vi "Compile Routing and Faulting Config.vi"(8 "error in (no error)":errorcluster, 11 "Device Ref in":T1 format="%.0x") -> (0 "error out":errorcluster, 2 "RaF Configuration":T2, 3 "Device Ref out":T1 format="%.0x")   [LabVIEW 2017, in "Routing and Faulting System Explorer.lvlib"]
uses:
  Routing and Faulting System Explorer.lvlib
  Shared/Routing and Faulting Configuration.ctl
  Shared/Routing Channel Configuration.ctl
  Shared/Value-Connections Map.ctl
  Shared/Connection.ctl
  <vilib>/NI Veristand/Custom Device API/Custom Device Item Ref.ctl
  Shared/Constants.vi
  <vilib>/NI Veristand/Custom Device Tools/Custom Device Utility Library/NI VeriStand - Search for Item by Name.vi
  Shared/Routing and Faulting Shared.lvlib
  <vilib>/NI Veristand/Custom Device Tools/Custom Device Utility Library/Custom Device Utility Library.lvlib
  Scripting/Switch Scripting.lvlib
  <vilib>/NI VeriStand/Custom Device API/Custom Device API.lvlib
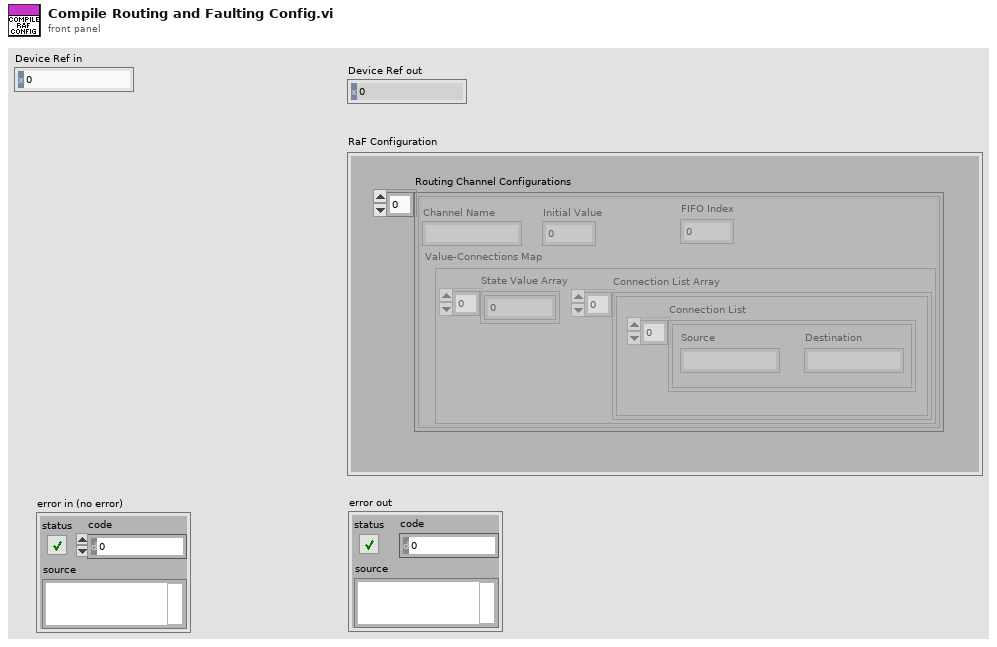
[diagram p1: front panel]
types:
  T1 = typedef "Custom Device API.lvlib/Custom Device Item Ref.ctl" = u64
  T2 = typedef "Routing and Faulting Shared.lvlib/Routing and Faulting Configuration.ctl" = cluster{"Routing Channel Configurations":T3[]}
  T3 = typedef "Routing and Faulting Shared.lvlib/Routing Channel Configuration.ctl" = cluster{"Channel Name":string, "Initial Value":dbl, "FIFO Index":i32, "Value-Connections Map":T4}
  T4 = typedef "Routing and Faulting Shared.lvlib/Value-Connections Map.ctl" = cluster{"State Value Array":i32[], "Connection List Array":cluster{"Connection List":T5[]}[]}
  T5 = typedef "Routing and Faulting Shared.lvlib/Connection.ctl" = cluster{"Source":string, "Destination":string}
  T6 = typedef "Routing and Faulting Shared.lvlib/Channel States.ctl" = T7[]
  T7 = typedef "Routing and Faulting Shared.lvlib/Routing State.ctl" = cluster{"Name":string, "Description":string, "Value":i32, "Connection List":T5[]}
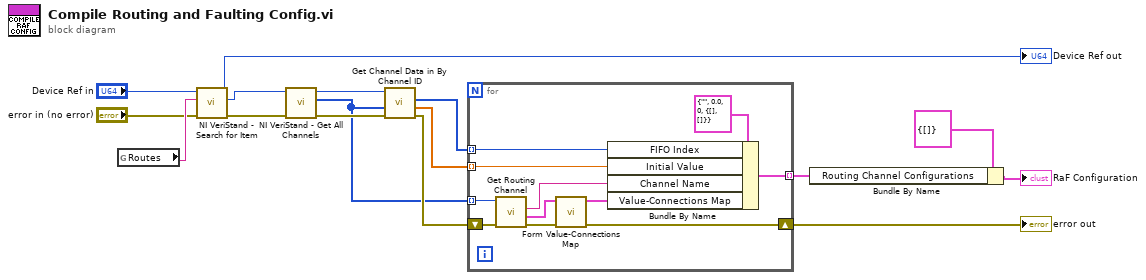
[diagram p0: block diagram]
diagram:
  n1 = global read "Constants.vi" "Routes"() -> (w14:string)
  n2 = call-poly <vilib>:"NI VeriStand - Search for Item.vi"("error in"="error in (no error)", "Item Name"=w14, "Section Ref in"="Device Ref in") -> ("error out"=w9:errorcluster, "Item Ref"=w10:T1, "Section Ref out"=→"Device Ref out":T1)  [unwired: 5 in, 1 out]
  n3 = call <vilib>:"NI VeriStand - Get All Channels.vi"("error in"=w9, "Section Ref in"=w10) -> ("error out"=w7:errorcluster, "Channel Refs"=w6:T1[], "Section Ref out"=w8:T1)  [unwired: 6 in, 1 out]
  n4 = call "Get Channel Data in By Channel ID.vi"("error in (no error)"=w7, "Channel IDs"=w6, "Section Ref in"=w8) -> ("error out"=w11:errorcluster, "default values"=w13:dbl[], "FIFO indexes"=w12:i32[])  [unwired: 4 in, 2 out]
  n5 = for {
    tunnel: w6 -> [w27] mode=indexing
    tunnel: w13 -> [w22] mode=indexing
    tunnel: w12 -> [w25] mode=indexing
    shift-right: [w19] -> w2
    shift-left: w11 -> [w23]
    tunnel: [w21] -> w5 mode=indexing
    n6 = call "Get Routing Channel.vi"("error in (no error)"=w23, "Channel Ref in"=w27) -> ("error out"=w20:errorcluster, "Channel States"=w18:T6, "Channel Name"=w24:string)  [unwired: 5 in, 2 out]
    n7 = call "Form Value-Connections Map.vi"("error in (no error)"=w20, "Channel States"=w18) -> ("error out"=w19:errorcluster, "Value-Connections Map"=w17:T4)  [unwired: 8 in]
    n8 = Bundle By Name(cluster=T3 {"Channel Name"="", "Initial Value"=0.0, "FIFO Index"=0, "Value-Connections Map"={"State Value Array"=[], "Connection List Array"=[]}} ("Routing Channel Configuration"), "FIFO Index"=w25, "Initial Value"=w22, "Channel Name"=w24, "Value-Connections Map"=w17) -> (w21:T3)
  }
  "error out" <- w2
  n9 = Bundle By Name(cluster=T2 {"Routing Channel Configurations"=[]} ("Routing and Faulting Configuration"), "Routing Channel Configurations"=w5) -> (→"RaF Configuration":T2)
